vi "Package Data.vi"(8 "error in (no error)":errorcluster, 10 "DataIn":string, 11 "VC Data in":refnum<class "VC Data.lvclass">) -> (0 "error out":errorcluster, 3 "VC Data out":refnum<class "VC Data.lvclass">)   [LabVIEW 2015, in "VC Data.lvclass"]
uses:
  VC Data.lvclass
  VC Data.lvclass/VC Data.ctl
  <vilib>/MSR Consulting, LLC/General Reuse/Data/Write measTime.vi
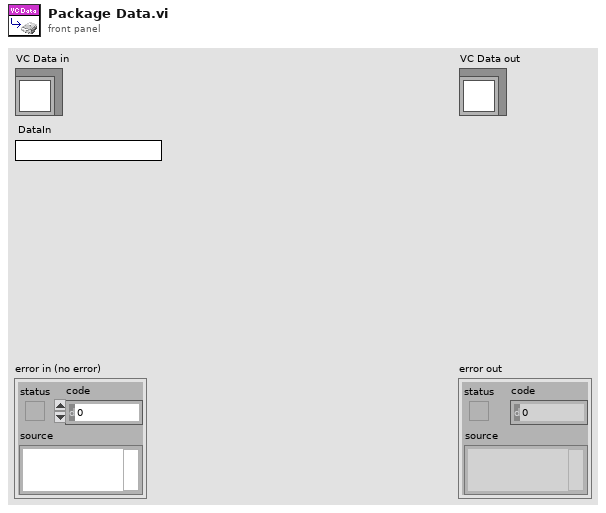
[diagram p1: front panel]
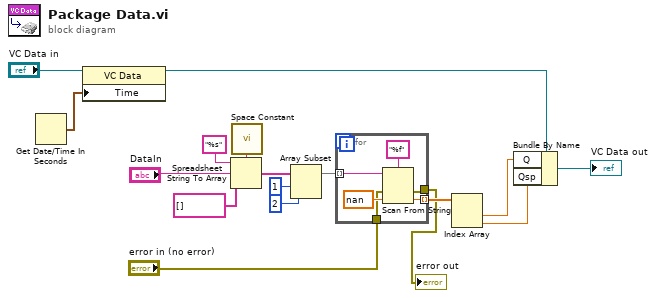
[diagram p0: block diagram]
diagram:
  n1 = Get Date/Time In Seconds() -> (seconds since 1Jan1904=w2:timestamp)
  n2 = property class="VC Data"(reference="VC Data in", "Time"=w2) -> (reference out=w6:refnum<class "VC Data.lvclass">)  [unwired: 1 in, 1 out]
  n3 = call <vilib>:"Space Constant.vi"() -> ("String"=w16:string)
  n4 = Spreadsheet String To Array(delimiter (Tab)=w16, format string="%s", spreadsheet string="DataIn", array type (2D Dbl)=string[] []) -> (array=w13:string[])
  n5 = Array Subset(array=w13, index=1, length=2) -> (w10:string[])
  n6 = for {
    tunnel: w10 -> [w23] mode=indexing
    tunnel: [w20] -> w14 mode=indexing
    tunnel: "error in (no error)" -> [w19]
    tunnel: [w18] -> w3
    n7 = Scan From String(format string="%f", input string=w23, error in=w19, default 1=sgl nan ("default value 1")) -> (error out=w18:errorcluster, output 1=w20:sgl)  [unwired: 1 in, 2 out]
  }
  "error out" <- w3
  n8 = Index Array(array=w14) -> (element #1=w5:sgl, element #2=w4:sgl)  [unwired: 2 in]
  n9 = Bundle By Name(cluster=w6, "Q"=w5, "Qsp"=w4) -> (→"VC Data out":refnum<class "VC Data.lvclass">)
